vi "Add Copyright to Folder.vi"(8 "error in (no error)":errorcluster, 9 "Type":T1={"vi"=TRUE, "ctl"=TRUE, "lvlib"=TRUE, "lvclass"=TRUE, "lvproj"=TRUE} caption="Select File Type to Add Copyright", 10 "Copyright Text":string="© Company Name", 11 "Source Code Directory":path) -> (0 "error out":errorcluster)   [LabVIEW 2016, in "SLL Add Copyright.lvlib"]
doc: "Add/update copyright text to all LabVIEW files in the provided folder. \n\nSupported LabVIEW files are *.vi, *.ctl, *.lvlib, *.lvclass and *.lvproj."
uses:
  SLL Add Copyright.lvlib
  _Typedefs/Select File Type.ctl
panel:
  out "Progress":i32(slide) scale=0.0..5.0
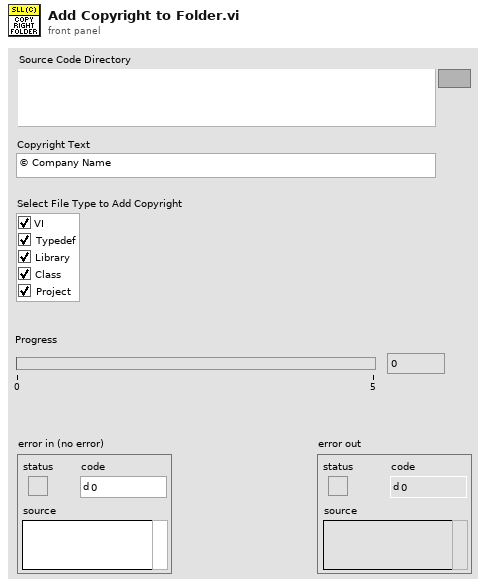
[diagram p1: front panel]
types:
  T1 = typedef "SLL Add Copyright.lvlib/Select File Type.ctl" = cluster{"vi":bool, "ctl":bool, "lvlib":bool, "lvclass":bool, "lvproj":bool}
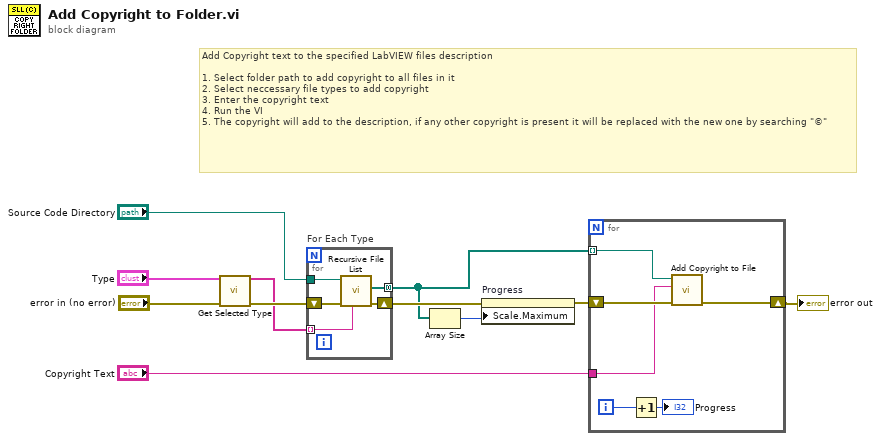
[diagram p0: block diagram]
diagram:
  # "Add Copyright text to the specified LabVIEW files description\n\n1. Select folder path to add copyright to all files in it\n2. Select neccessary file types to add copyright\n3. Enter the copyright text\n4. Run the VI\n5. The copyright will add to the description, if any other copyright is present it will be replaced with the new one by searching \"©\""
  n1 = call "Get Selected Type.vi"("Select Type"="Type", "error in (no error)"="error in (no error)") -> ("Selected File Types[]"=w6:string[], "error out"=w9:errorcluster)  [unwired: 12 in]
  n2 = for "For Each Type" {
    tunnel: "Source Code Directory" -> [w14]
    tunnel: w6 -> [w13] mode=indexing
    tunnel: [w12] -> w5 mode=concatenating
    shift-right: [w15] -> w8
    shift-left: w9 -> [w16]
    n3 = call <vilib>:"Recursive File List.vi"("pattern"=w13, "error in (no error)"=w16, "Folder Path"=w14) -> ("error out"=w15:errorcluster, "All Files in Dir"=w12:path[])  [unwired: 4 in, 3 out]
  }
  n4 = Array Size(array=w5) -> (size(s)=w4:i32)
  n5 = property on="Progress" class="Slide (strict)"(error in=w8, "Scale.Maximum"=w4) -> (error out=w10:errorcluster)  [unwired: 1 in, 1 out]
  n6 = for {
    shift-right: [w20] -> w2
    shift-left: w10 -> [w21]
    tunnel: w5 -> [w22] mode=indexing
    tunnel: "Copyright Text" -> [w17]
    i -> [w19]
    n7 = Increment(x=w19) -> (x+1=→"Progress":i32)
    n8 = call "Add Copyright to File.vi"("error in (no error)"=w21, "Copyright Text"=w17, "File Path"=w22) -> ("error out"=w20:errorcluster)  [unwired: 8 in]
  }
  "error out" <- w2
